vi "jsonToString.vi"(7 "pretty print?":bool, 8 "error in (no error)":errorcluster, 10 "path":string, 11 "d in":i64) -> (0 "error out":errorcluster, 2 "json string":string, 3 "d out":i64)   [LabVIEW 2015, in "rapidjson wrapper.lvlib"]
uses:
  rapidjson wrapper.lvlib
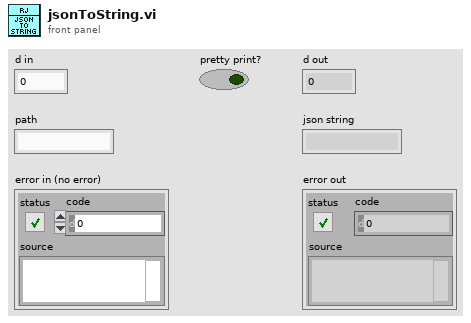
[diagram p1: front panel]
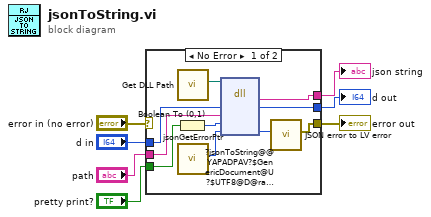
[diagram p0: block diagram]
diagram:
  n1 = case shown="No Error" "error in (no error)" {
    selector: "error in (no error)" -> [_ w19]
    tunnel: [w15 _] -> w7
    tunnel: [w14 w18] -> w6
    tunnel: "d in" -> [w13 w18]
    tunnel: "path" -> [w12 _]
    tunnel: [w10 w19] -> w3
    tunnel: "pretty print?" -> [w8 _]
    frame No Error {
      n2 = Boolean To (0,1)(Boolean=w8) -> (0, 1=w9:i16)
      n3 = call "Get DLL Path.vi"() -> ("Path"=w17:path)  [unwired: 11 in]
      n4 = call "jsonGetErrorPtr.vi"() -> ("return type"=w16:i64)  [unwired: 10 in, 1 out]
      n5 = dll-call lib="C:/Users/tblair/Documents/Git Projects/rapidjson-for-LabVIEW/lvrjs/Debug/lvrjs.dll" fn="?jsonToString@@YAPADPAV?$GenericDocument@U?$UTF8@D@rapidjson@@V?$MemoryPoolAllocator@VCrtAllocator@rapidjson@@@2@VCrtAllocator@2@@rapidjson@@PAD_N0@Z"(path in=w17, "d"=w13, "path"=w12, "prettyPrint"=w9, "jsonError"=w16) -> ("return type"=w15:string, "d"=w14:i64, "jsonError"=w11:i64)  [unwired: 4 in, 2 out]
      n6 = call "JSON error to LV error.vi"("jsonError"=w11) -> ("error out"=w10:errorcluster)  [unwired: 10 in]
    }
    frame Error {
    }
  }
  "json string" <- w7
  "d out" <- w6
  "error out" <- w3
